vi "Group Page GUID.vi"() -> (3 "Group GUID":string="473b4065-4cef-436d-b68a-ef19370f2b9b")   [LabVIEW 2021, in "DSF Shared.lvlib"]
uses:
  DSF Shared.lvlib
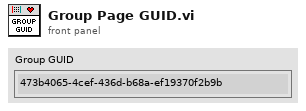
[diagram p1: front panel]
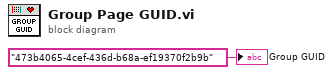
[diagram p0: block diagram]
diagram:
  "Group GUID" <- "473b4065-4cef-436d-b68a-ef19370f2b9b" ("Data Sharing Framework")
